vi "SubVI_Read_Write_EEG_Acc.vi"(8 "error in (no error)":errorcluster, 10 "Weight Array":i32[](array[numeric]), 11 "LINX Resource in":T2) -> (0 "error out":errorcluster, 1 "Raw EEG":T1, 2 "LINX Resource out":T2, 3 "Acc Data Out":T1)   [LabVIEW 2020]
uses:
  <vilib>/MakerHub/LINX/Private/Type Defs/LINX Ref.ctl
  <vilib>/MakerHub/LINX/Private/Type Defs/Platform.ctl
  <vilib>/MakerHub/LINX/Private/Type Defs/Interface.ctl
  <vilib>/MakerHub/LINX/Private/Device/Type Defs/LINX Device Config.ctl
  <vilib>/MakerHub/LINX/Private/Device/Type Defs/TCP Config.ctl
  <vilib>/MakerHub/LINX/Private/Device/Type Defs/Channels.ctl
  <extravilib>/ChannelInstances/Lossy Stream-a[.](dbl)/)Channel.ctl
  <vilib>/MakerHub/LINX/Private/Type Defs/Peripherals/SPI/SPI Configuration.ctl
  <vilib>/MakerHub/LINX/Private/Type Defs/Peripherals/SPI/SPI Bit Order.ctl
  <vilib>/MakerHub/LINX/Private/Type Defs/Peripherals/SPI/SPI Mode.ctl
  <vilib>/MakerHub/LINX/Public/Peripherals/SPI/SPI CS Config.ctl
  <vilib>/MakerHub/LINX/Private/Type Defs/Peripherals/SPI/SPI CS Logic Level.ctl
  <vilib>/MakerHub/LINX/Public/Peripherals/SPI/SPI Write Read 1 Frame.vi
  <vilib>/MakerHub/LINX/Public/Peripherals/SPI/SPI Write Read N Frames.vi
  <extravilib>/ChannelInstances/Lossy Stream-a[.](dbl)/Endpoint.vi
  <vilib>/MakerHub/LINX/Private/Local IO/LinxSpiWriteRead.vi
  <vilib>/MakerHub/LINX/Public/Utilities/Check Channel.vi
  <vilib>/MakerHub/LINX/Private/Local IO/Handle Errors.vi
  Global 1.vi
  <vilib>/MakerHub/LINX/Private/Utilties/Generate Error.vi
  <extravilib>/ChannelInstances/Lossy Stream-a[.](dbl)/)Channel.vi
  <vilib>/MakerHub/LINX/LMH-LINX.lvlib
  <extravilib>/ChannelInstances/Lossy Stream-a[.](dbl).lvlib
  <vilib>/MakerHub/LINX/Private/Device/Device.lvlib
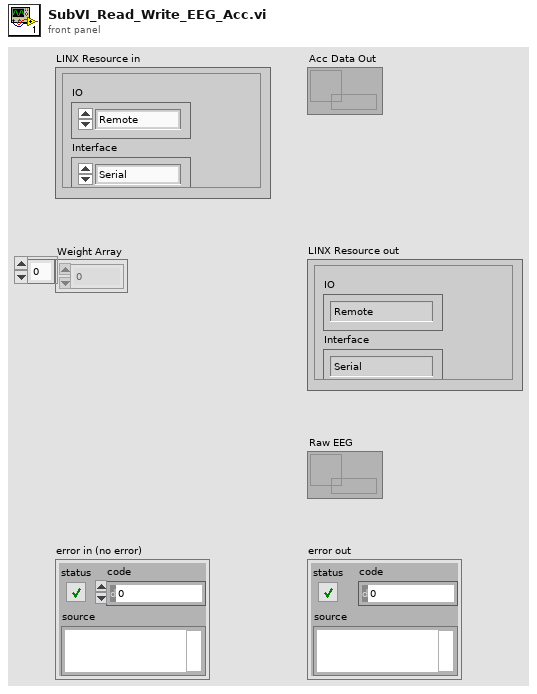
[diagram p1: front panel]
types:
  T1 = typedef "Lossy Stream-a[.](dbl).lvlib/)Channel.ctl" = refnum<queue>
  T2 = typedef "LMH-LINX.lvlib/LINX Ref.ctl" = cluster{"IO":T3, "Interface":T4, "LINX Device Config":T5}
  T3 = typedef "LMH-LINX.lvlib/Platform.ctl" = enum16{"Remote", "Local"}
  T4 = typedef "LMH-LINX.lvlib/Interface.ctl" = enum16{"Serial", "TCP"}
  T5 = typedef "LMH-LINX.lvlib/Device.lvlib/LINX Device Config.ctl" = cluster{"Interface":T4, "COM Port":refnum<visa-resource-name>, "TCP Configuration":T6, "Device Family":u8, "Device ID":u8, "Device Name":string, "TCP Ref":refnum<k5>, "Channels":T7}
  T6 = typedef "LMH-LINX.lvlib/Device.lvlib/TCP Config.ctl" = cluster{"IP Address":string, "Port":u16}
  T7 = typedef "LMH-LINX.lvlib/Channels.ctl" = cluster{"DI":u8[], "DO":u8[], "AI":u8[], "AO":u8[], "PWM":u8[], "QE":u8[], "UART":u8[], "I2C 2":u8[], "SPI":u8[], "CAN":u8[], "Servo":u8[], "AI Ref (V)":dbl, "AI Resolution (Bits)":u8, "AO Ref (V)":dbl, "AO Resolution (Bits)":u8}
  T8 = typedef "LMH-LINX.lvlib/SPI CS Config.ctl" = cluster{"CS Channel":u8, "CS Logic Level":T9}
  T9 = typedef "LMH-LINX.lvlib/SPI CS Logic Level.ctl" = enum8{"Active Low", "Active High"}
  T10 = typedef "LMH-LINX.lvlib/SPI Configuration.ctl" = cluster{"Clock Frequency":u32, "Bit Order":T11, "SPI Mode":T12}
  T11 = typedef "LMH-LINX.lvlib/SPI Bit Order.ctl" = enum8{"LSb First", "MSb First"}
  T12 = typedef "LMH-LINX.lvlib/SPI Mode.ctl" = enum8{"Mode 0", "Mode 1", "Mode 2", "Mode 3"}
  T13 = typedef "LVDateTimeRec.ctl" = cluster{"fractional second":dbl, "second":i32, "minute":i32, "hour":i32, "day of month":i32, "month":i32, "year":i32, "day of week":i32, "day of year":i32, "DST":i32}
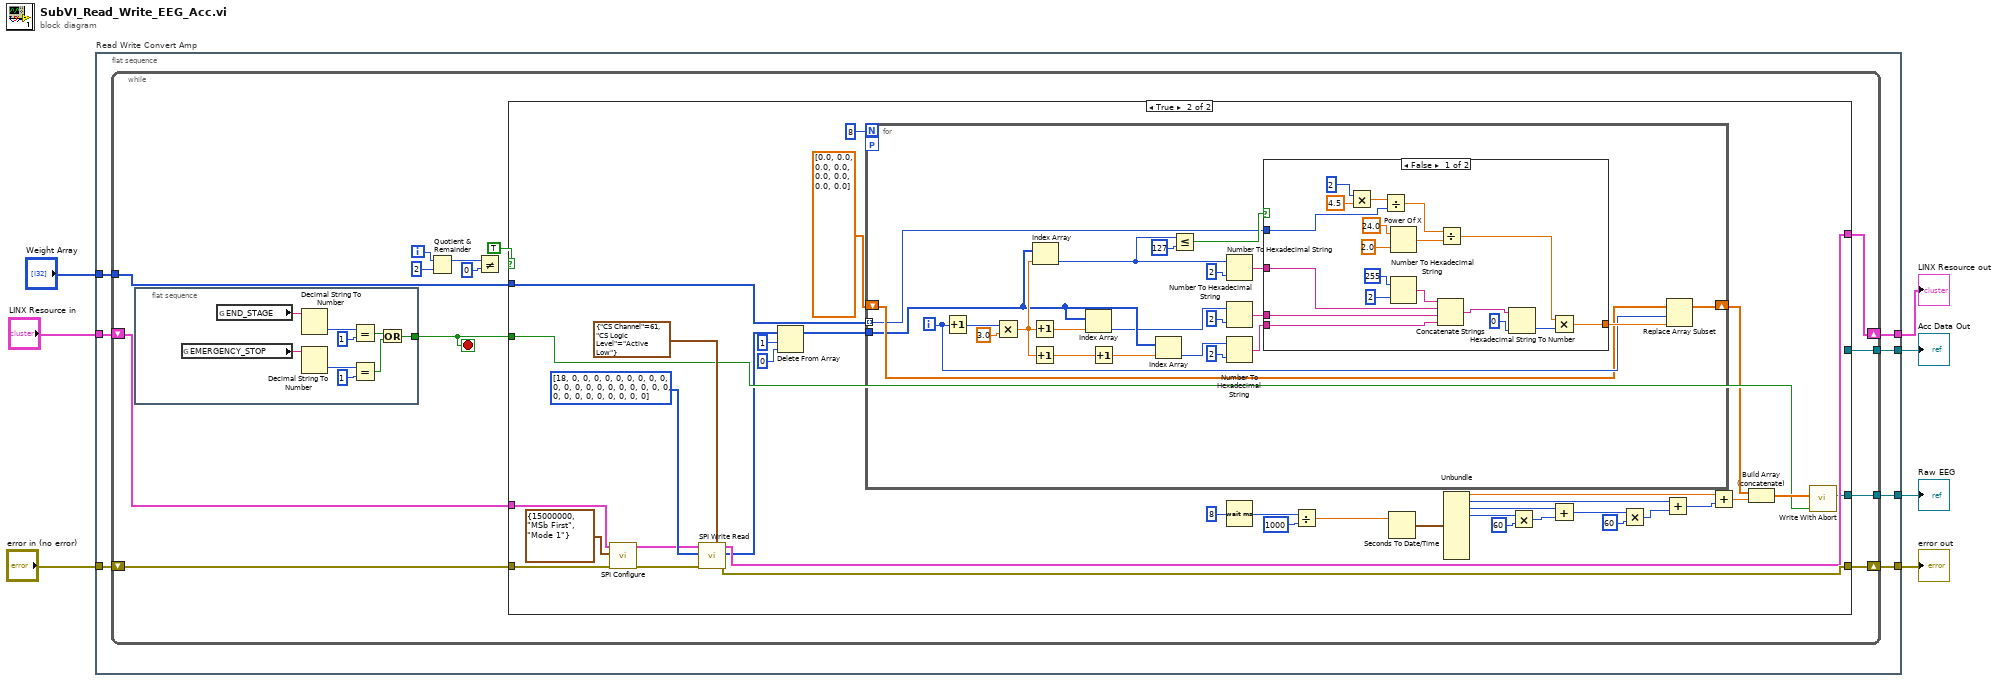
[diagram p0: block diagram]
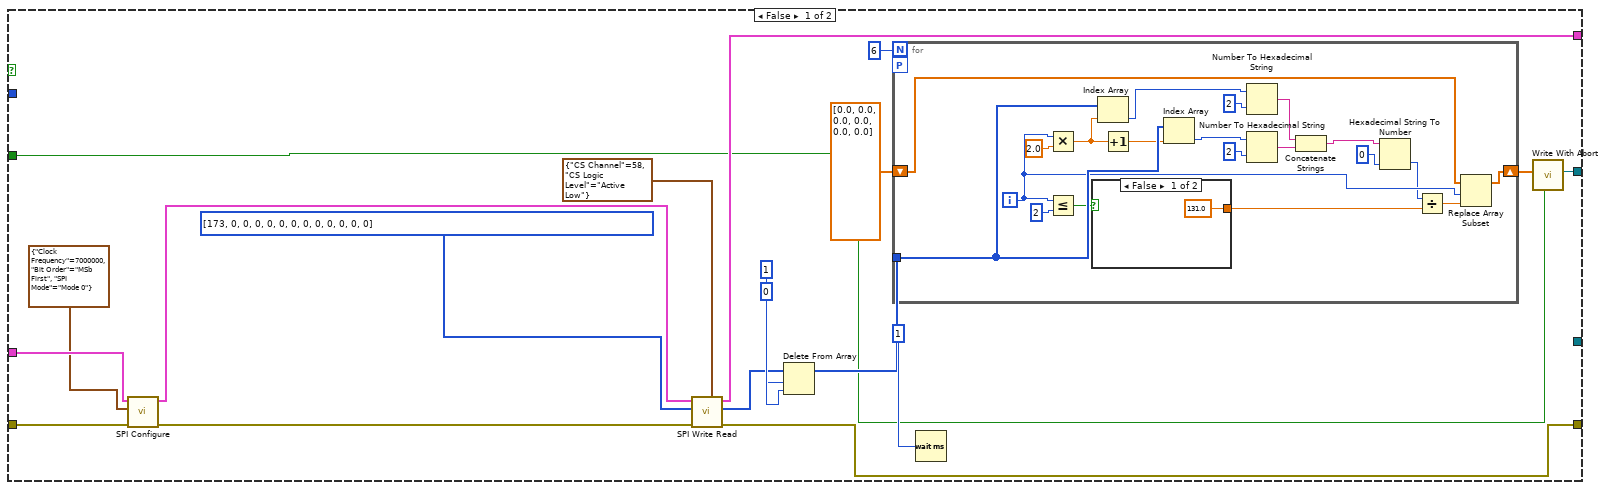
[diagram p2: hidden frame]
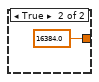
[diagram p3: hidden frame]
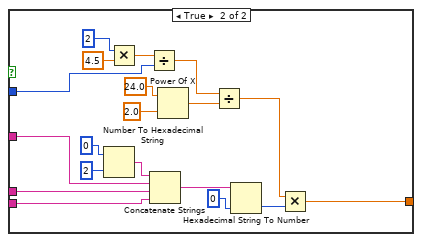
[diagram p4: hidden frame]
diagram:
  n1 = flat-sequence "Read Write Convert Amp" {
    tunnel: [w14] -> w5
    tunnel: [w13] -> w1
    tunnel: [w12] -> w2
    tunnel: "error in (no error)" -> [w11]
    tunnel: "LINX Resource in" -> [w10]
    tunnel: "Weight Array" -> [w9]
    tunnel: [w8] -> w4
    frame #0 {
      n2 = while {
        shift-right: [w22] -> w13
        shift-left: w11 -> [w21]
        shift-right: [w20] -> w14
        shift-left: w10 -> [w23]
        tunnel: [w19] -> w12
        tunnel: w9 -> [w18]
        tunnel: [w17] -> w8
        i -> [w27]
        stop <- w16 stop-if-true
        n3 = flat-sequence {
          tunnel: [w28] -> w16
          frame #0 {
            n4 = global read "Global 1.vi" "EMERGENCY_STOP"() -> (w31:string)
            n5 = global read "Global 1.vi" "END_STAGE"() -> (w36:string)
            n6 = Decimal String To Number(string=w36) -> (number=w35:i32)  [unwired: 2 in, 1 out]
            n7 = Decimal String To Number(string=w31) -> (number=w33:i32)  [unwired: 2 in, 1 out]
            n8 = Equal?(x=w35, y=1) -> (x = y?=w29:bool)
            n9 = Equal?(x=w33, y=1) -> (x = y?=w30:bool)
            n10 = Or(x=w29, y=w30) -> (x .or. y?=w28:bool)
          }
        }
        n11 = Quotient & Remainder(x=w27, y=2) -> (x-y*floor(x/y)=w25:i32)  [unwired: 1 out]
        n12 = Not Equal?(x=w25, y=0) -> ()  [unwired: 1 out]
        n13 = case shown="True" TRUE {
          tunnel: w23 -> [w54 w113]
          tunnel: [w50 w111] -> w22
          tunnel: w21 -> [w55 w110]
          tunnel: [w49 w109] -> w20
          tunnel: w16 -> [w37 w87]
          tunnel: [_ w88] -> w19
          tunnel: w18 -> [_ w82]
          tunnel: [w38 _] -> w17
          frame False {
            n14 = call <vilib>:"SPI Configure.vi"("Error In"=w55, "SPI Configuration"=T10 {"Clock Frequency"=7000000, "Bit Order"=enum."MSb First", "SPI Mode"=enum."Mode 0"}, "LINX Resource"=w54) -> ("Error Out"=w48:errorcluster, "LINX Resource"=w47:T2)  [unwired: 6 in, 1 out]
            n15 = call-poly <vilib>:"SPI Write Read.vi"("CS Configuration"=T8 {"CS Channel"=58, "CS Logic Level"=enum."Active Low"}, "Error In"=w48, "Data"=u8[] [173, 0, 0, 0, 0, 0, 0, 0, 0, 0, 0, 0, 0], "LINX Resource"=w47) -> ("Error Out"=w50:errorcluster, "Read Data"=w41:u8[], "LINX Resource"=w49:T2)  [unwired: 4 in, 1 out]
            n16 = Delete From Array(array=w41, length=1, index=0) -> (array with subset deleted=w40:u8[])  [unwired: 1 out]
            n17 = for {
              N: 6 -> [_]
              shift-right: [w73] -> w39
              shift-left: dbl[] [0.0, 0.0, 0.0, 0.0, 0.0, 0.0] -> [w74]
              tunnel: w40 -> [w72]
              workers-P: _ -> [_]
              i -> [w71]
              n18 = Multiply(x=w71, y=2.0) -> (x*y=w64:dbl)
              n19 = Less Or Equal?(x=w71, y=2) -> (x <= y?=w57:bool)
              n20 = case shown="False" w57 {
                tunnel: [131.0 ("y") 16384.0 ("y")] -> w56
                frame False {
                }
                frame True {
                }
              }
              n21 = Index Array(array=w72, index=w64) -> (element=w61:u8)
              n22 = Increment(x=w64) -> (x+1=w63:dbl)
              n23 = Index Array(array=w72, index=w63) -> (element=w62:u8)
              n24 = Number To Hexadecimal String(1:i16 2 ("width (-)"), 2:w61) -> (0:w68:string)
              n25 = Number To Hexadecimal String(1:i16 2 ("width (-)"), 2:w62) -> (0:w69:string)
              n26 = Concatenate Strings(w68, w69) -> (w60:string)
              n27 = Hexadecimal String To Number(string=w60, default (0uL)=i16 0 ("default (0 U32)")) -> (number=w58:i16)  [unwired: 1 in, 1 out]
              n28 = Divide(x=w58, y=w56) -> (x/y=w75:dbl)
              n29 = Replace Array Subset(array=w74, new element=w75, index=w71) -> (w73:dbl[])
            }
            n30 = Wait (ms)(milliseconds to wait=u32 1) -> ()  [unwired: 1 out]
            n31 = call <extravilib>:"Write With Abort.vi"("abort"=w37, "element"=w39) -> ("channel"=w38:T1)  [unwired: 6 in, 3 out]
          }
          frame True {
            n32 = call <vilib>:"SPI Configure.vi"("Error In"=w110, "SPI Configuration"=T10 {"Clock Frequency"=15000000, "Bit Order"=enum."MSb First", "SPI Mode"=enum."Mode 1"}, "LINX Resource"=w113) -> ("Error Out"=w106:errorcluster, "LINX Resource"=w105:T2)  [unwired: 6 in, 1 out]
            n33 = call-poly <vilib>:"SPI Write Read.vi"("CS Configuration"=T8 {"CS Channel"=61, "CS Logic Level"=enum."Active Low"}, "Error In"=w106, "Data"=u8[] [18, 0, 0, 0, 0, 0, 0, 0, 0, 0, 0, 0, 0, 0, 0, 0, 0, 0, 0, 0, 0, 0, 0, 0, 0, 0, 0, 0, 0, 0], "LINX Resource"=w105) -> ("Error Out"=w111:errorcluster, "Read Data"=w84:u8[], "LINX Resource"=w109:T2)  [unwired: 4 in, 1 out]
            n34 = Delete From Array(array=w84, length=1, index=0) -> (array with subset deleted=w83:u8[])  [unwired: 1 out]
            n35 = for {
              N: 8 -> [_]
              shift-right: [w119] -> w79
              shift-left: dbl[] [0.0, 0.0, 0.0, 0.0, 0.0, 0.0, 0.0, 0.0] -> [w120]
              tunnel: w83 -> [w117]
              tunnel: w82 -> [w118] mode=indexing
              workers-P: _ -> [_]
              i -> [w121]
              n36 = Increment(x=w121) -> (x+1=w127:i32)
              n37 = Multiply(x=w127, y=3.0) -> (x*y=w126:dbl)
              n38 = Increment(x=w126) -> (x+1=w123:dbl)
              n39 = Increment(x=w126) -> (x+1=w124:dbl)
              n40 = Index Array(array=w117, index=w126) -> (element=w114:u8)
              n41 = Index Array(array=w117, index=w123) -> (element=w115:u8)
              n42 = Increment(x=w124) -> (x+1=w125:dbl)
              n43 = Index Array(array=w117, index=w125) -> (element=w116:u8)
              n44 = Less Or Equal?(x=w114, y=u8 127) -> (x <= y?=w135:bool)
              n45 = Number To Hexadecimal String(1:i16 2 ("width (-)"), 2:w114) -> (0:w132:string)
              n46 = Number To Hexadecimal String(1:i16 2 ("width (-)"), 2:w115) -> (0:w133:string)
              n47 = Number To Hexadecimal String(1:i16 2 ("width (-)"), 2:w116) -> (0:w134:string)
              n48 = case shown="False" w135 {
                tunnel: w134 -> [w146 w164]
                tunnel: w133 -> [w147 w163]
                tunnel: w132 -> [w148 w162]
                tunnel: [w142 w161] -> w122
                tunnel: w118 -> [w137 w156]
                frame False {
                  n49 = Multiply(x=2, y=4.5) -> (x*y=w153:dbl)
                  n50 = Divide(x=w153, y=w137) -> (x/y=w150:dbl)
                  n51 = Power Of X(1:2.0 ("x"), 2:24.0 ("y")) -> (0:w149:dbl)
                  n52 = Number To Hexadecimal String(1:i16 2 ("width (-)"), 2:255) -> (0:w144:string)
                  n53 = Concatenate Strings(w144, w148, w147, w146) -> (w140:string)
                  n54 = Divide(x=w150, y=w149) -> (x/y=w143:dbl)
                  n55 = Hexadecimal String To Number(string=w140, default (0uL)=0 ("default (0 U32)")) -> (number=w139:i32)  [unwired: 1 in, 1 out]
                  n56 = Multiply(x=w143, y=w139) -> (x*y=w142:dbl)
                }
                frame True {
                  n57 = Number To Hexadecimal String(1:i16 2 ("width (-)"), 2:0) -> (0:w166:string)
                  n58 = Multiply(x=2, y=4.5) -> (x*y=w172:dbl)
                  n59 = Divide(x=w172, y=w156) -> (x/y=w169:dbl)
                  n60 = Concatenate Strings(w166, w162, w163, w164) -> (w159:string)
                  n61 = Power Of X(1:2.0 ("x"), 2:24.0 ("y")) -> (0:w168:dbl)
                  n62 = Divide(x=w169, y=w168) -> (x/y=w165:dbl)
                  n63 = Hexadecimal String To Number(string=w159, default (0uL)=0 ("default (0 U32)")) -> (number=w160:i32)  [unwired: 1 in, 1 out]
                  n64 = Multiply(x=w165, y=w160) -> (x*y=w161:dbl)
                }
              }
              n65 = Replace Array Subset(array=w120, new element=w122, index=w121) -> (w119:dbl[])
            }
            n66 = Wait (ms)(milliseconds to wait=u32 8) -> (millisecond timer value=w101:u32)
            n67 = Divide(x=w101, y=u32 1000) -> (x/y=w102:dbl)
            n68 = Seconds To Date/Time(time stamp (now)=w102) -> (date time rec=w100:T13)  [unwired: 1 in]
            n69 = Unbundle(w100) -> ("fractional second"=w90:dbl, "second"=w91:i32, "minute"=w93:i32, "hour"=w95:i32)  [unwired: 6 out]
            n70 = Multiply(x=w95, y=60) -> (x*y=w99:i32)
            n71 = Add(x=w93, y=w99) -> (x+y=w98:i32)
            n72 = Multiply(x=w98, y=60) -> (x*y=w97:i32)
            n73 = Add(x=w91, y=w97) -> (x+y=w96:i32)
            n74 = Add(x=w90, y=w96) -> (x+y=w78:dbl)
            n75 = Build Array (concatenate)(w79, w78) -> (w89:dbl[])
            n76 = call <extravilib>:"Write With Abort.vi"("abort"=w87, "element"=w89) -> ("channel"=w88:T1)  [unwired: 6 in, 3 out]
          }
        }
      }
    }
  }
  "LINX Resource out" <- w5
  "Acc Data Out" <- w4
  "Raw EEG" <- w2
  "error out" <- w1
